vi "Init 5761.vi"(6 "Record length":u16, 8 "error in (no error)":errorcluster, 9 "Mode":T1, 10 "Clock Source":T3, 11 "FPGA ref":T2) -> (0 "error out":errorcluster, 3 "FpgaRef5761 out":refnum<class "FpgaRef5761.lvclass">)   [LabVIEW 2013, in "FpgaRef5761.lvclass"]
uses:
  FpgaRef5761.lvclass
  ClockSource_5761.ctl
  5761 FPGA ref.ctl
  FPGA/DataMode.ctl
  FpgaRef5761.lvclass/FpgaRef5761.ctl
  <vilib>/rvi/interface/common/niFpgaWaitOnOcc.vi
  <vilib>/Utility/error.llb/Error Cluster From Error Code.vi
  <vilib>/rvi/errors/niLvFpgaAdjustHostInterfaceError.vi
  <vilib>/rvi/interface/nirviReadWriteControl/nirviReadWriteControl.xnode
  NiFpgaLv.dll
  <vilib>/rvi/interface/Simulation/niFpgaSimulationCallBeginRW.vi
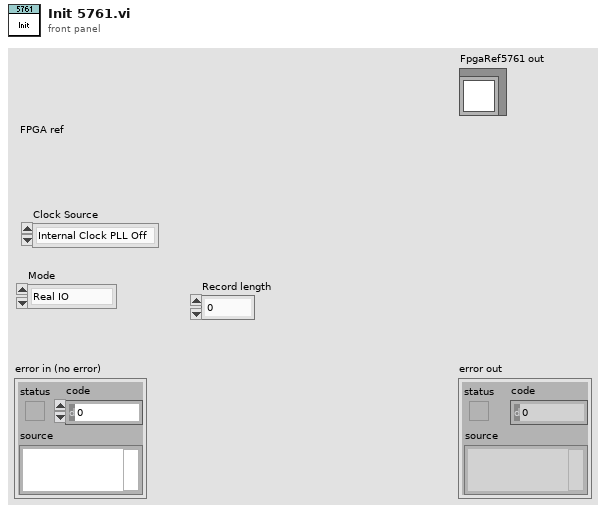
[diagram p1: front panel]
types:
  T1 = typedef "DataMode.ctl" = enum16{"Real IO", "Simulated"}
  T2 = typedef "5761 FPGA ref.ctl" = refnum<k20>
  T3 = typedef "ClockSource_5761.ctl" = enum8{"Internal Clock PLL Off", "Internal Clock PLL On (CLK_IN)", "External Clock (CLK_IN)", "Internal Clock PLL On (IoModSyncClk)", "External Clock (IoModSyncClk)"}
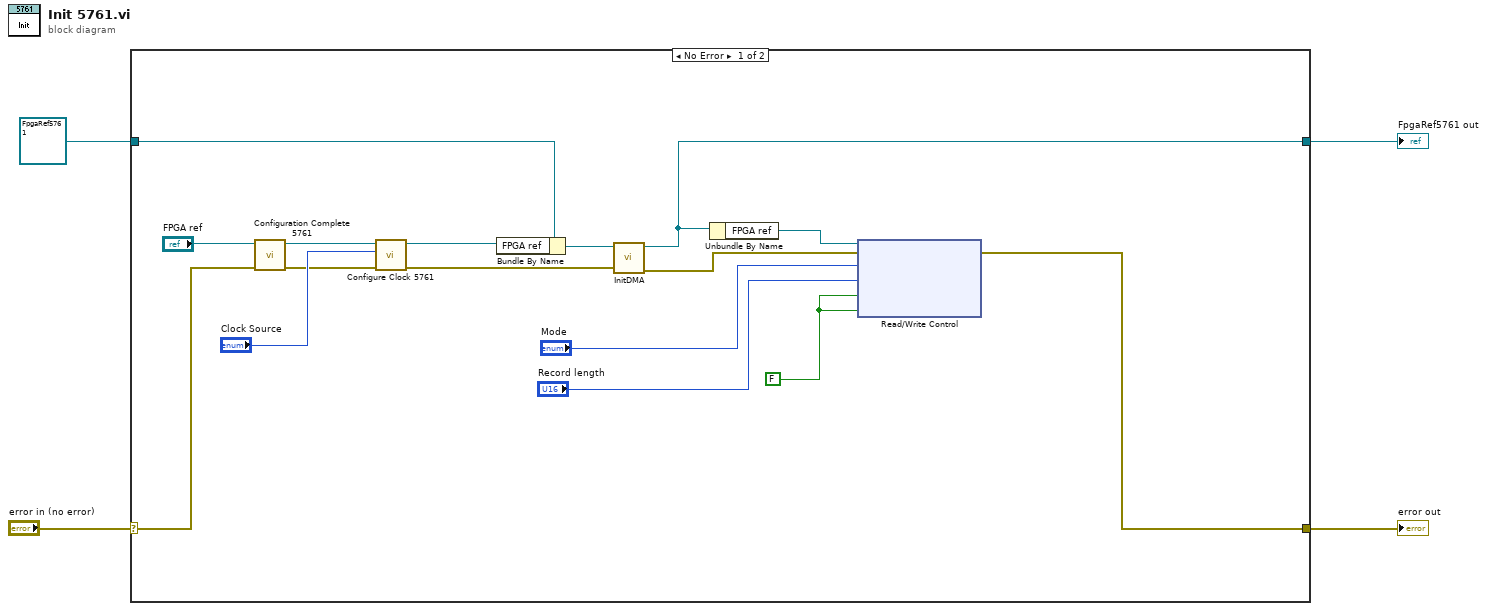
[diagram p0: block diagram]
diagram:
  n1 = case shown="No Error" "error in (no error)" {
    selector: "error in (no error)" -> [w13 w22]
    tunnel: [w5 w22] -> w3
    tunnel: [w10 w21] -> w2
    tunnel: refnum<class "FpgaRef5761.lvclass"> refnum ("FpgaRef5761 in") -> [w12 w21]
    frame No Error {
      w11 = FALSE
      n2 = call "Configuration Complete 5761.vi"("error in"=w13, "FPGA Interface"="FPGA ref") -> ("error out"=w15:errorcluster, "FPGA VI Reference Out"=w20:T2)  [unwired: 7 in, 1 out]
      n3 = call "Configure Clock 5761.vi"("error in"=w15, "Clock Source"="Clock Source", "FPGA Interface"=w20) -> ("error out"=w14:errorcluster, "FPGA VI Reference Out"=w17:T2)  [unwired: 6 in, 1 out]
      n4 = Bundle By Name(cluster=w12, "FPGA ref"=w17) -> (w16:refnum<class "FpgaRef5761.lvclass">)
      n5 = call-dynamic "InitDMA.vi"("error in (no error)"=w14, "FpgaRef5761 in"=w16) -> ("error out"=w6:errorcluster, "FpgaRef5761 out"=w10:refnum<class "FpgaRef5761.lvclass">)  [unwired: 8 in]
      n6 = Unbundle By Name(w10) -> ("FPGA ref"=w9:T2)
      n7 = xnode "Read/Write Control"("FPGA VI Reference In"=w9, "error in"=w6, "Mode"="Mode", "5782 record length"="Record length", "Trigger Acquisition"=w11, "Acquisition running"=w11) -> ("error out"=w5:errorcluster)  [unwired: 1 out]
    }
    frame Error {
    }
  }
  "error out" <- w3
  "FpgaRef5761 out" <- w2
